vi "BRig_dataExp_Audio_pattern_1B.vi"() -> (2 "output_Audio_sp__1B":i32)   [LabVIEW 2014]
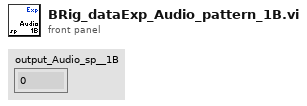
[diagram p1: front panel]
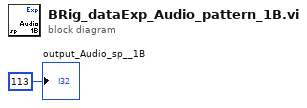
[diagram p0: block diagram]
diagram:
  "output_Audio_sp__1B" <- 113 ("output_iBlock")
